vi "Universal B-I-V.vi"() -> ()   [LabVIEW 2021]
panel:
  in  "error in (no error)":errorcluster
  in  "Tab Control":enum32{"Log", "Module Choose", "Range"}(tab)
  in  "folder":bool
  in  "File Name":string="Sample"
  in  "base path":path=path "C:/Users/gyue/Box Sync/Guang Yue/data"
  out "Generated File name":string
  in  "Book number":i32=357
  in  "Magnet Control":enum32{"None", "Elsa 5T", "Keithley 2400"}(tab)=enum."Keithley 2400"
  in  "Book Number":i32
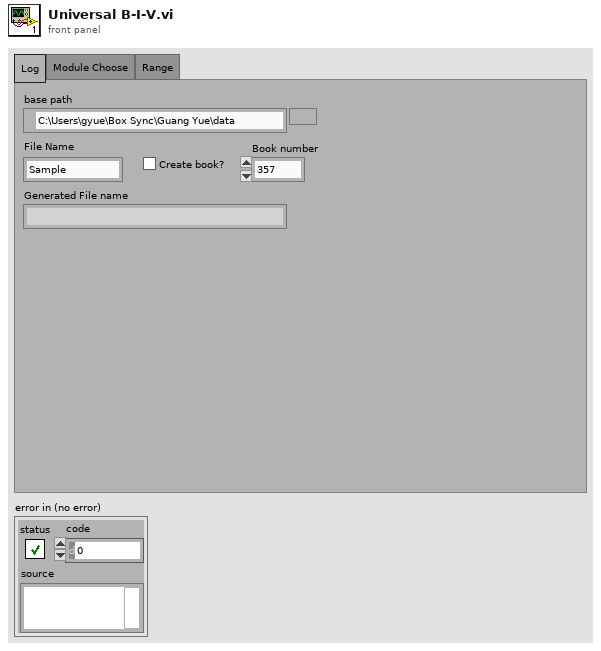
[diagram p1: front panel]
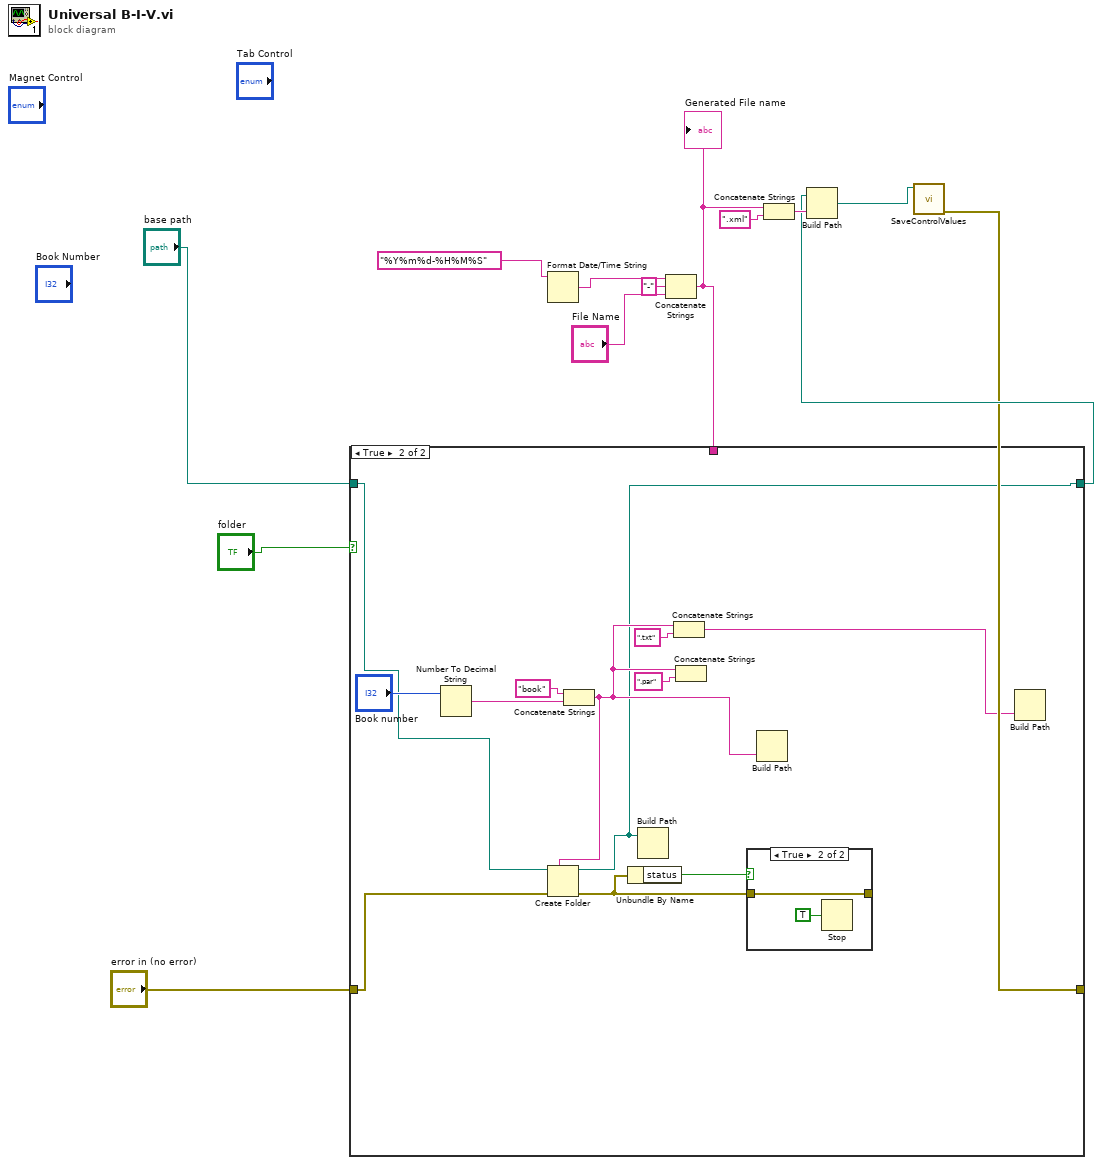
[diagram p0: block diagram]
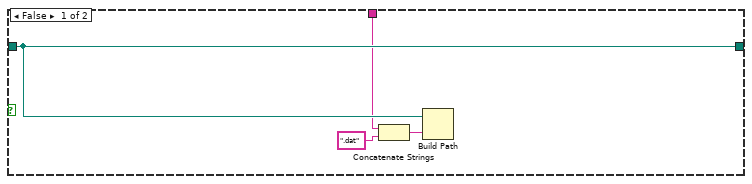
[diagram p2: hidden frame]
diagram:
  n1 = Format Date/Time String(time format string (%c)="%Y%m%d-%H%M%S") -> (date/time string=w12:string)  [unwired: 2 in]
  n2 = Concatenate Strings(w12, "-" ("string"), "File Name") -> (w3:string)
  "Generated File name" <- w3
  n3 = case shown="True" "folder" {
    tunnel: "base path" -> [w17 w21]
    tunnel: [w17 w19] -> w4
    tunnel: w3 -> [w15 _]
    tunnel: "error in (no error)" -> [_ w18]
    tunnel: [_ _] -> w1
    frame False {
      n4 = Concatenate Strings(w15, ".dat" ("string")) -> (w16:string)
      n5 = Build Path(base path=w17, name or relative path=w16) -> ()  [unwired: 1 out]
    }
    frame True {
      n6 = Number To Decimal String(number="Book number") -> (decimal integer string=w29:string)  [unwired: 1 in]
      n7 = Concatenate Strings("book" ("string"), w29) -> (w20:string)
      n8 = Create Folder(prompt (Create Folder)=w20, path (use dialog)=w21, error in=w18) -> (created path=w19:path, error out=w23:errorcluster)  [unwired: 1 out]
      n9 = Unbundle By Name(w23) -> ("status"=w22:bool)
      n10 = Build Path(base path=w19) -> ()  [unwired: 1 in, 1 out]
      n11 = Concatenate Strings(w20, ".txt" ("string")) -> (w27:string)
      n12 = Concatenate Strings(w20, ".par" ("string")) -> ()  [unwired: 1 out]
      n13 = case shown="True" w22 {
        tunnel: [w30 w32] -> _
        tunnel: w23 -> [w30 w32]
        frame False {
        }
        frame True {
          n14 = Stop(stop? (T)=TRUE) -> ()
        }
      }
      n15 = Build Path(name or relative path=w20) -> ()  [unwired: 1 in, 1 out]
      n16 = Build Path(name or relative path=w27) -> ()  [unwired: 1 in, 1 out]
    }
  }
  n17 = Concatenate Strings(w3, ".xml" ("string")) -> (w11:string)
  n18 = Build Path(base path=w4, name or relative path=w11) -> (appended path=w10:path)
  n19 = call "SaveControlValues.vi"("XML File Path"=w10, "error in (no error)"=w1) -> ()  [unwired: 8 in, 1 out]
